vi "lift setpoints final.vi"(7 "Set Motor Speed":dbl=0.25, 11 "Requested Position\n(0, 1, 2, 4, 8, 16)":i32=16) -> (1 "Setpoint\nReached":bool, 3 "Motor Speed":dbl)   [LabVIEW 2014]
uses:
  Global Variables/Sensor Data (Edited).vi
  Global Variables/Settings.vi
  Global Variables/Miscalleneous.vi
panel:
  out "Requested Position":i32=16
  out "Current Position":i32
  # "0 is when none of the \npositions are Called\n1, is when Lift Position one has been called\n2, is  whn lift position two has been called\n4 is when lift position three has been called\n8, is when lift position four has been called\n16 is when lift position five has been called"
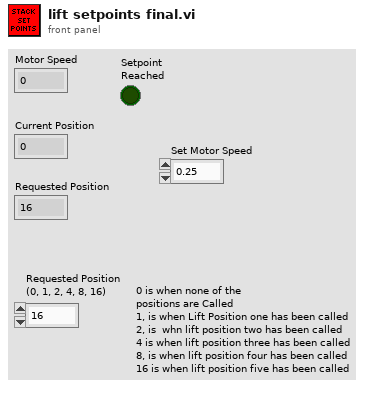
[diagram p1: front panel]
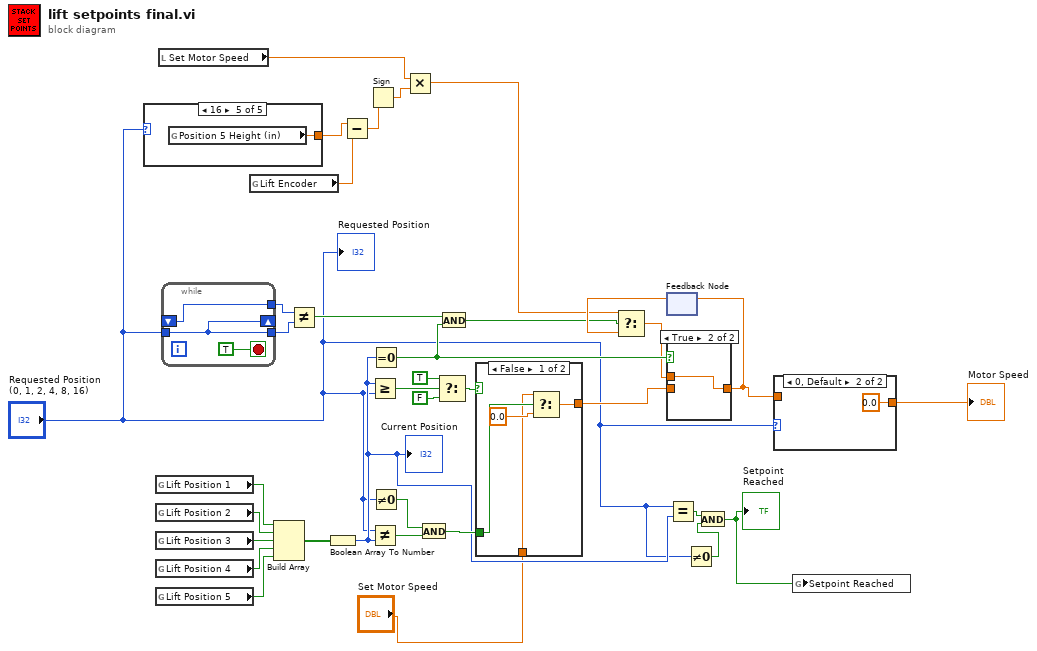
[diagram p0: block diagram]
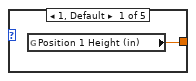
[diagram p2: hidden frame]
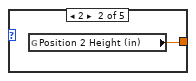
[diagram p3: hidden frame]
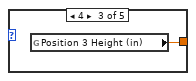
[diagram p4: hidden frame]
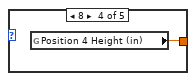
[diagram p5: hidden frame]
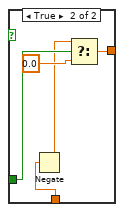
[diagram p8: hidden frame]
diagram:
  n1 = case shown="16" "Requested Position\n(0, 1, 2, 4, 8, 16)" {
    tunnel: [w36 w37 w38 w39 w40] -> w6
    frame 1, Default {
      n2 = global read "Settings.vi" "Position 1 Height (in)"() -> (w36:dbl)
    }
    frame 2 {
      n3 = global read "Settings.vi" "Position 2 Height (in)"() -> (w37:dbl)
    }
    frame 4 {
      n4 = global read "Settings.vi" "Position 3 Height (in)"() -> (w38:dbl)
    }
    frame 8 {
      n5 = global read "Settings.vi" "Position 4 Height (in)"() -> (w39:dbl)
    }
    frame 16 {
      n6 = global read "Settings.vi" "Position 5 Height (in)"() -> (w40:dbl)
    }
  }
  n7 = global read "Sensor Data (Edited).vi" "Lift Position 1"() -> (w22:bool)
  n8 = global read "Sensor Data (Edited).vi" "Lift Position 2"() -> (w23:bool)
  n9 = global read "Sensor Data (Edited).vi" "Lift Position 3"() -> (w24:bool)
  n10 = global read "Sensor Data (Edited).vi" "Lift Position 4"() -> (w25:bool)
  n11 = global read "Sensor Data (Edited).vi" "Lift Position 5"() -> (w26:bool)
  n12 = local read "Set Motor Speed"() -> (w8:dbl)
  n13 = while {
    tunnel: "Requested Position\n(0, 1, 2, 4, 8, 16)" -> [w42]
    tunnel: [w42] -> w17
    shift-right: [w42] -> _
    shift-left: _ -> [w41]
    tunnel: [w41] -> w16
    stop <- TRUE stop-if-true
  }
  n14 = global read "Sensor Data (Edited).vi" "Lift Encoder"() -> (w5:dbl)
  n15 = Build Array(w22, w23, w24, w25, w26) -> (w32:bool[])
  n16 = Not Equal?(x=w16, y=w17) -> (x != y?=w15:bool)
  n17 = Boolean Array To Number(Boolean array=w32) -> (number=w21:u32)
  "Current Position" <- w21
  n18 = Subtract(x=w6, y=w5) -> (x-y=w10:dbl)
  n19 = Sign(1:w10) -> (0:w9:dbl)
  n20 = Greater Or Equal?(x=w21, y="Requested Position\n(0, 1, 2, 4, 8, 16)") -> (x >= y?=w31:bool)
  n21 = Not Equal?(x="Requested Position\n(0, 1, 2, 4, 8, 16)", y=w21) -> (x != y?=w30:bool)
  n22 = Equal To 0?(x=w21) -> (x = 0?=w14:bool)
  n23 = Not Equal To 0?(x="Requested Position\n(0, 1, 2, 4, 8, 16)") -> (x != 0?=w29:bool)
  n24 = Multiply(x=w8, y=w9) -> (x*y=w7:dbl)
  n25 = And(x=w29, y=w30) -> (x .and. y?=w28:bool)
  n26 = Select(t=TRUE, s=w31, f=FALSE) -> (s? t:f=w33:bool)
  n27 = And(x=w15, y=w14) -> (x .and. y?=w12:bool)
  n28 = case shown="False" w33 {
    tunnel: w28 -> [w46 w51]
    tunnel: [w45 w50] -> w27
    tunnel: "Set Motor Speed" -> [w44 w49]
    frame False {
      n29 = Select(t=w44, s=w46, f=0.0) -> (s? t:f=w45:dbl)
    }
    frame True {
      n30 = Negate(x=w49) -> (-x=w48:dbl)
      n31 = Select(t=w48, s=w51, f=0.0) -> (s? t:f=w50:dbl)
    }
  }
  n32 = feedback #1() -> (w13:dbl)  [unwired: 1 in]
  n33 = Select(t=w7, s=w12, f=w13) -> (s? t:f=w11:dbl)
  n34 = case shown="True" w14 {
    tunnel: w27 -> [w53 _]
    tunnel: [w53 w54] -> w18
    tunnel: w11 -> [_ w54]
    frame False {
    }
    frame True {
    }
  }
  n35 = feedback-in #1(w18) -> ()
  n36 = Equal?(x="Requested Position\n(0, 1, 2, 4, 8, 16)", y=w21) -> (x = y?=w3:bool)
  n37 = Not Equal To 0?(x="Requested Position\n(0, 1, 2, 4, 8, 16)") -> (x != 0?=w2:bool)
  n38 = And(x=w3, y=w2) -> (x .and. y?=w4:bool)
  "Setpoint\nReached" <- w4
  n39 = case shown="0, Default" "Requested Position\n(0, 1, 2, 4, 8, 16)" {
    tunnel: [w55 0.0 ("Set Motor Speed")] -> w19
    tunnel: w18 -> [w55 _]
    frame 1, 2, 4, 8, 16 {
    }
    frame 0, Default {
    }
  }
  "Motor Speed" <- w19
  n40 = global write "Miscalleneous.vi" "Setpoint Reached"(w4) -> ()
  "Requested Position" <- "Requested Position\n(0, 1, 2, 4, 8, 16)"
